vi "AdaptToInputs.vi"(3 "Term Types":T1[](array[typedef]), 4 "XRef":refnum<vi>, 5 "State In":T4) -> (0 "Reply":string[](array[string]), 2 "State Out":T4)   [LabVIEW 2012, in "CRefScripting.lvlib" / "CRef Label Node.xnode"]
doc: "This ability VI is called by LabVIEW during type propagation so that your XNode may adapt itself to new input types. Term Types is an array of pairs of current Term IDs and the type descriptors corresponding to them. The type descriptors are taken from the signal connected to the terminal. Unwired terminals are not included in the array. Use Reply to inform LabVIEW of any actions it needs to take.\n\nDefault behavior: None.\n\nThis ability does not provide UI and OS messages are not handled."
uses:
  CRef Label Node.xnode
  State.ctl
  Core/Master Types.ctl
  <vilib>/XNodeSupport/XNodeTermTypeIDPair.ctl
  <vilib>/XNodeSupport/XNodeType.ctl
  <vilib>/XNodeSupport/XNodeString.ctl
  <vilib>/XNodeSupport/NI_XNodeSupport.lvlib
  CRef.lvlib
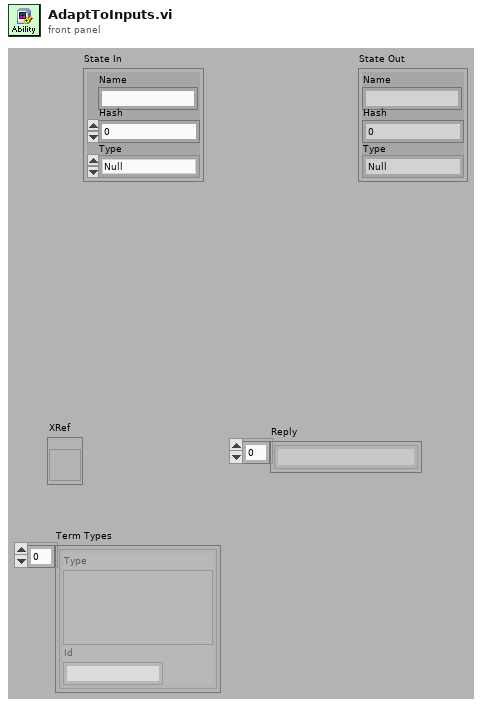
[diagram p1: front panel]
types:
  T1 = typedef "NI_XNodeSupport.lvlib/XNodeTermTypeIDPair.ctl" = cluster{"Type":T2, "Id":T3}
  T2 = typedef "NI_XNodeSupport.lvlib/XNodeType.ctl" = variant
  T3 = typedef "NI_XNodeSupport.lvlib/XNodeString.ctl" = string
  T4 = typedef "CRefScripting.lvlib/CRef Label Node.xnode/State.ctl" = cluster{"Name":string, "Hash":u32, "Type":T5}
  T5 = typedef "CRef.lvlib/Master Types.ctl" = enum8{"Null", "Boolean", "U8", "I8", "U16", "I16", "U32", "I32", "U64", "I64", "Single", "Double", "Extended", "CSG", "CDB", "CXT", "Boolean(Def)", "U8(Def)", "I8(Def)", "U16(Def)", "I16(Def)", "U32(Def)", "I32(Def)", "Reserved Def", "Reserved Def1", "Single(Def)", "Double(Def)", "Reserved Def2", "Reserved Def3", "Reserved Def4", "Reserved Def5", "Unsigned(Def)", "Signed(Def)", "Real(Def)", "Reserved Def6", "Numeric(Def)", "String"}
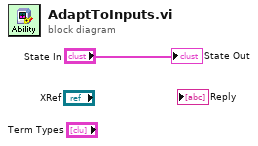
[diagram p0: block diagram]
diagram:
  "State Out" <- "State In"
